vi "Fetch Measurement (Channel Power).vi"(0 "VISA resource name":refnum<visa-resource-name>, 11 "error in (no error)":errorcluster) -> (4 "VISA resource name out":refnum<visa-resource-name>, 6 "Channel Power(dBm/Integrated BW MHz)":dbl, 10 "Channel Power Density(dBm/Hz)":dbl, 15 "error out":errorcluster)   [LabVIEW 2022 SP3, in "Agilent N934X Series.lvlib"]
doc: "Returns the results of last measurement (Channel Power) and does not initiate data acquisition.\n\nNote:\n\nThis VI does not check the instrument status. Typically, you call this VI only in a sequence of calls to other low-level instrument driver VIs. The sequence performs one operation. You use the low-level VIs to optimize one or more aspects of interaction with the instrument. If you want to check the instrument status, call the <B>Error Query VI</B> at the conclusion of the sequence."
uses:
  <instrlib>/Agilent N934X Series/Agilent N934X Series.lvlib
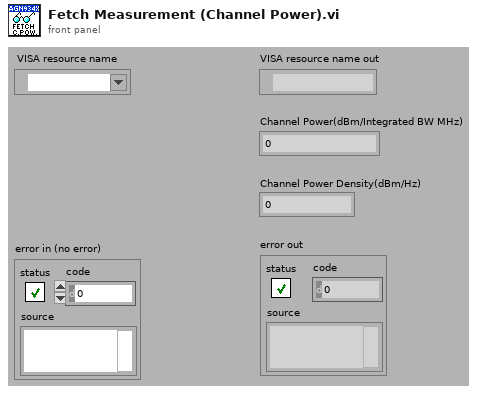
[diagram p1: front panel]
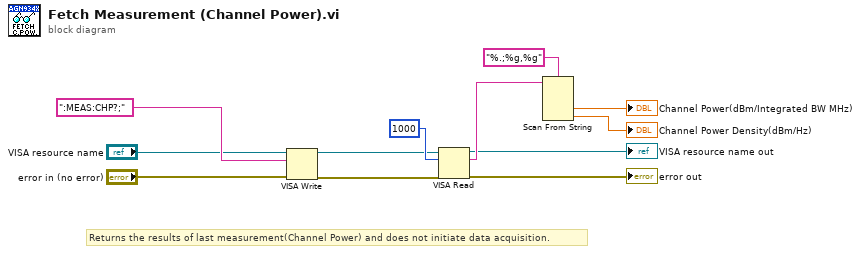
[diagram p0: block diagram]
diagram:
  # "Returns the results of last measurement(Channel Power) and does not initiate data acquisition."
  n1 = VISA Write(VISA resource name="VISA resource name", write buffer=":MEAS:CHP?;", error in (no error)="error in (no error)") -> (VISA resource name out=w8:refnum<visa-resource-name>, error out=w7:errorcluster)  [unwired: 1 out]
  n2 = VISA Read(VISA resource name=w8, byte count=u32 1000, error in (no error)=w7) -> (VISA resource name out=→"VISA resource name out":refnum<visa-resource-name>, read buffer=w6:string, error out=→"error out":errorcluster)  [unwired: 1 out]
  n3 = Scan From String(format string="%.;%g,%g", input string=w6) -> (output 1=→"Channel Power(dBm/Integrated BW MHz)":dbl, output 2=→"Channel Power Density(dBm/Hz)":dbl)  [unwired: 4 in, 3 out]
